vi "ToRepo.vi"(8 "error in":errorcluster, 9 "to repo cluster":T1, 10 "repository in":refnum<class "NISE_CEF_Repository.lvclass">, 11 "node in":refnum<class "Dependencies.lvclass">) -> (0 "error out":errorcluster, 2 "repository out":refnum<class "NISE_CEF_Repository.lvclass">, 3 "node out":refnum<class "Dependencies.lvclass">)   [LabVIEW 2015, in "Dependencies.lvclass"]
doc: "Transfers the information from the tree node into the repo. How it is stored in the repo depends on the Repo.Copyright 2015 National Instruments Corporation\n\nLicensed under the Apache License, Version 2.0 (the \"License\"); you may not use this file except in compliance with the License. You may obtain a copy of the License at http://www.apache.org/licenses/LICENSE-2.0\nUnless required by applicable law or agreed to in writing, software distributed under the License is distributed on an \"AS IS\" BASIS, WITHOUT WARRANTIES OR CONDITIONS OF ANY KIND, either express or implied. See the License for the specific language governing permissions and limitations under the License."
uses:
  Dependencies.lvclass
  <vilib>/NI/Configuration Framework/Repository/NISE_CEF_Repository.lvclass
  <vilib>/NI/Configuration Framework/Node/ToRepoCluster.ctl
  CustomDeviceRepo/CustomDeviceRepo.lvclass
  Dependencies.lvclass/Dependencies.ctl
  <vilib>/NI/Configuration Framework/Node/NISE_CEF_Node.lvclass
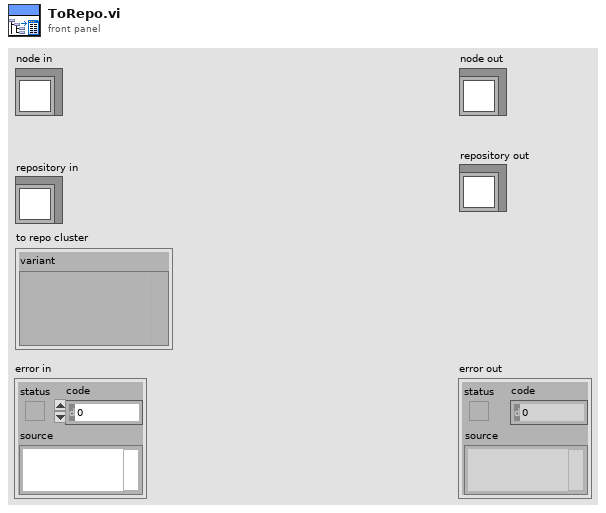
[diagram p1: front panel]
types:
  T1 = typedef "NISE_CEF_Node.lvclass/ToRepoCluster.ctl" = cluster{"variant":variant}
  T2 = typedef "VeriStand Custom Device XML Parser.lvlib/Dependencies Properties.ctl" = cluster{"ForceDownload":bool, "RealTimeSystemDestination":string, "Path Properties":T3, "Supported Target":T4, "Version":string, "SupportedTargetSpecified":bool}
  T3 = typedef "VeriStand Custom Device XML Parser.lvlib/Path Cluster.ctl" = cluster{"Path":path, "Path Type":enum16{"Absolute", "To Base", "To Common Doc Dir", "To Application Data Dir"}}
  T4 = typedef "VeriStand Custom Device XML Parser.lvlib/Supported Targets.ctl" = enum16{"All", "Pharlap", "VxWorks", "Windows", "Linux_32_ARM", "Linux_x64", "PharlapWindows", "PharlapVxWorks", "VxWorksWindows"}
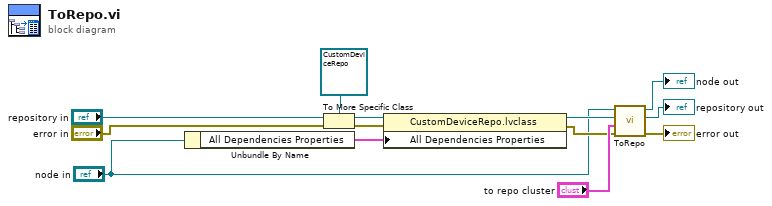
[diagram p0: block diagram]
diagram:
  n1 = Unbundle By Name("node in") -> ("All Dependencies Properties"=w6:T2[])
  n2 = To More Specific Class(target class=refnum<class "CustomDeviceRepo.lvclass"> refnum ("CustomDeviceRepo.lvclass"), reference="repository in", error in="error in") -> (specific class reference=w10:refnum<class "CustomDeviceRepo.lvclass">, error out=w9:errorcluster)
  n3 = property class="CustomDeviceRepo.lvclass"(reference=w10, error in=w9, "All Dependencies Properties"=w6) -> (reference out=w7:refnum<class "CustomDeviceRepo.lvclass">, error out=w3:errorcluster)
  n4 = call-parent "ToRepo.vi"("error in"=w3, "to repo cluster"="to repo cluster", "repository in"=w7, "node in"="node in") -> ("error out"=→"error out":errorcluster, "repository out"=→"repository out":refnum<class "NISE_CEF_Repository.lvclass">, "node out"=→"node out":refnum<class "Dependencies.lvclass">)  [unwired: 5 in]
